vi "Edit Chassis.vi"(8 "error in (no error)":errorcluster, 9 "Settings":T1={"Name"="", "Master Chassis"={"Type"=enum."None", "DAQ Name"="", "clkSrc"=10280, "activeEdge"=0, "exportClk"=0, "exportClkToLine"=0, "triggerLine"=10171, "triggerSlope"=0, "startTrigger"=0, "startTriggerLine"=0}} {"Master Chassis"."startTriggerLine" items=["None", "PFI_0", "PFI_1", "PFI_2", "PFI_3", "PFI_4", "PFI_5", "PFI_6", "PFI_7", "PFI_8", "PFI_9", "PFI_10", "PFI_11", "PFI_12", "PFI_13", "PFI_14", "PFI_15", "RTSI_PXI_TRIG_0", "RTSI_PXI_TRIG_1", "RTSI_PXI_TRIG_2", "RTSI_PXI_TRIG_3", "RTSI_PXI_TRIG_4", "RTSI_PXI_TRIG_5", "RTSI_PXI_TRIG_6", "RTSI_PXI_TRIG_7"]; "Master Chassis"."startTrigger" items=["aiStartTrigger", "aoStartTrigger"]; "Master Chassis"."triggerSlope" items=["Falling"=10171, "Rising"=10280]; "Master Chassis"."triggerLine" items=["None", "PFI_0", "PFI_1", "PFI_2", "PFI_3", "PFI_4", "PFI_5", "PFI_6", "PFI_7", "PFI_8", "PFI_9", "PFI_10", "PFI_11", "PFI_12", "PFI_13", "PFI_14", "PFI_15", "RTSI_PXI_TRIG_0", "RTSI_PXI_TRIG_1", "RTSI_PXI_TRIG_2", "RTSI_PXI_TRIG_3", "RTSI_PXI_TRIG_4", "RTSI_PXI_TRIG_5", "RTSI_PXI_TRIG_6", "RTSI_PXI_TRIG_7"]; "Master Chassis"."exportClkToLine" items=["Default_RTSI_PXI_TRIG_0", "PFI_0", "PFI_1", "PFI_2", "PFI_3", "PFI_4", "PFI_5", "PFI_6", "PFI_7", "PFI_8", "PFI_9", "PFI_10", "PFI_11", "PFI_12", "PFI_13", "PFI_14", "PFI_15", "RTSI_PXI_TRIG_0", "RTSI_PXI_TRIG_1", "RTSI_PXI_TRIG_2", "RTSI_PXI_TRIG_3", "RTSI_PXI_TRIG_4", "RTSI_PXI_TRIG_5", "RTSI_PXI_TRIG_6", "RTSI_PXI_TRIG_7"]; "Master Chassis"."exportClk" items=["aiSampleClock", "aoSampleClock"]; "Master Chassis"."activeEdge" items=["Falling"=10171, "Rising"=10280]; "Master Chassis"."clkSrc" items=["Onboard10MHzClock", "PFI_0", "PFI_1", "PFI_2", "PFI_3", "PFI_4", "PFI_5", "PFI_6", "PFI_7", "PFI_8", "PFI_9", "PFI_10", "PFI_11", "PFI_12", "PFI_13", "PFI_14", "PFI_15", "RTSI_PXI_TRIG_0", "RTSI_PXI_TRIG_1", "RTSI_PXI_TRIG_2", "RTSI_PXI_TRIG_3", "RTSI_PXI_TRIG_4", "RTSI_PXI_TRIG_5", "RTSI_PXI_TRIG_6", "RTSI_PXI_TRIG_7"]}, 10 "System Definition Node Path":string, 11 "SysDef Ref":T4) -> (0 "error out":errorcluster, 2 "New Node Path":string, 3 "SysDef Ref Out":T4)   [LabVIEW 2019, in "Simple SysDef API.lvlib"]
uses:
  <userlib>/SimpleSysDef/Simple SysDef API.lvlib
  <userlib>/SimpleSysDef/_SubVIs/System Definition Reference.ctl
  NationalInstruments.VeriStand.SystemDefinitionAPI
  <userlib>/SimpleSysDef/_SubVIs/Edit Chassis_Settings.ctl
  <userlib>/SimpleSysDef/_SubVIs/Add Chassis_DAQ Master Settings.ctl
  <userlib>/SimpleSysDef/_SubVIs/Add Chassis_Type.ctl
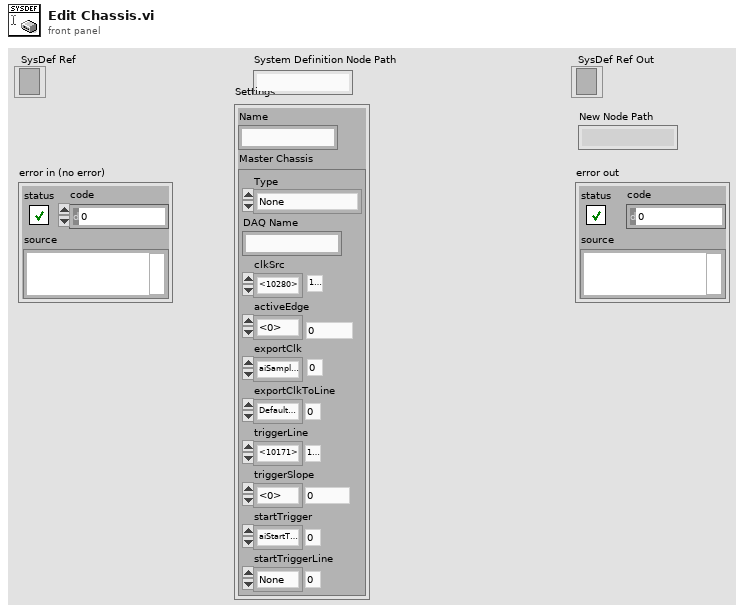
[diagram p1: front panel]
types:
  T1 = typedef "Simple SysDef API.lvlib/Edit Chassis_Settings.ctl" = cluster{"Name":string, "Master Chassis":T2}
  T2 = typedef "Simple SysDef API.lvlib/Add Chassis_DAQ Master Settings.ctl" = cluster{"Type":T3, "DAQ Name":string, "clkSrc":i32, "activeEdge":i32, "exportClk":i32, "exportClkToLine":i32, "triggerLine":i32, "triggerSlope":i32, "startTrigger":i32, "startTriggerLine":i32}
  T3 = typedef "Simple SysDef API.lvlib/Add Chassis_Type.ctl" = enum16{"None", "DAQ", "FPGA", "Timing and Sync", "Automatic"}
  T4 = typedef "Simple SysDef API.lvlib/System Definition Reference.ctl" = refnum<k24>
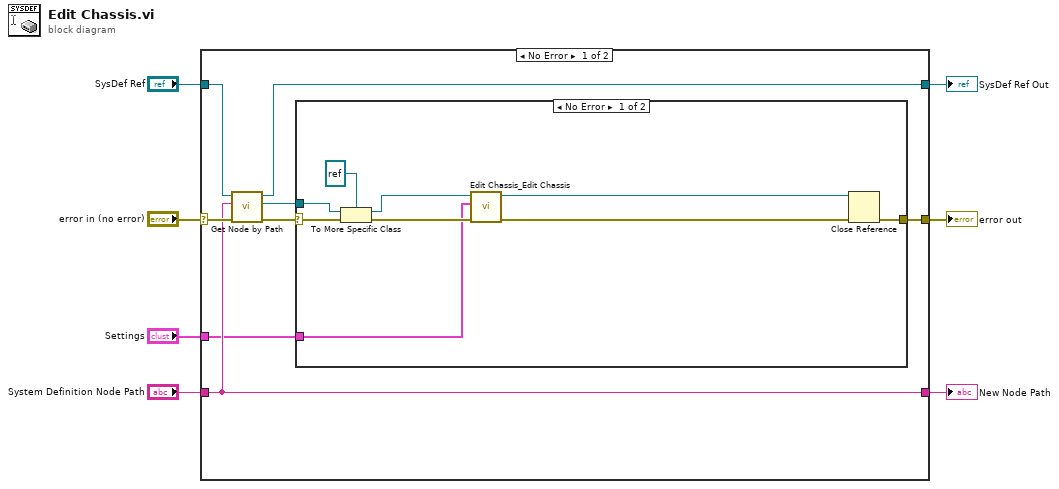
[diagram p0: block diagram]
diagram:
  n1 = case shown="No Error" "error in (no error)" {
    selector: "error in (no error)" -> [w15 w27]
    tunnel: [w12 w27] -> w6
    tunnel: "SysDef Ref" -> [w14 w26]
    tunnel: [w13 w26] -> w4
    tunnel: "System Definition Node Path" -> [w9 _]
    tunnel: "Settings" -> [w8 _]
    tunnel: [w9 _] -> w1
    frame No Error {
      n2 = call <userlib>:"Get Node by Path.vi"("error in (no error)"=w15, "System Definition Node Path"=w9, "SysDef Ref"=w14) -> ("error out"=w10:errorcluster, "Node Ref"=w11:refnum<k24>, "SysDef Ref Out"=w13:T4)  [unwired: 6 in]
      n3 = case shown="No Error" w10 {
        selector: w10 -> [w23 w25]
        tunnel: [w22 w25] -> w12
        tunnel: w11 -> [w24 _]
        tunnel: w8 -> [w16 _]
        frame No Error {
          n4 = To More Specific Class(target class=refnum<k24> refnum ("Node Ref"), reference=w24, error in=w23) -> (specific class reference=w18:refnum<k24>, error out=w20:errorcluster)
          n5 = call <userlib>:"Edit Chassis_Edit Chassis.vi"("error in (no error)"=w20, "Settings"=w16, "Chassis Ref"=w18) -> ("error out"=w19:errorcluster, "Chassis Ref Out"=w17:refnum<k24>)  [unwired: 7 in]
          n6 = Close Reference(reference=w17, error in (no error)=w19) -> (error out=w22:errorcluster)
        }
        frame Error {
        }
      }
    }
    frame Error {
    }
  }
  "SysDef Ref Out" <- w4
  "error out" <- w6
  "New Node Path" <- w1
